vi "ModeMgr.Init.vi"(6 "Default Config File":path=path "C:/MTE/Facility/Modes.json", 8 "error in (no error)":errorcluster, 9 "ControlRef":refnum<vi>, 10 "Config File":path=path "C:/MTE/Facility/Modes.json", 11 "ModeMgr In":refnum<class "Mode Manager.lvclass">) -> (0 "error out":errorcluster, 1 "Mode Settings":T1[](array[typedef]), 2 "Mode":string, 3 "ModeMgr Out":refnum<class "Mode Manager.lvclass">)   [LabVIEW 2018, in "Mode Manager.lvclass"]
uses:
  Mode Manager.lvclass
  ModeMgr.Mode Settings.ctl
  Mode Manager.lvclass/Mode Manager.ctl
  <vilib>/KATE/Files/File Utils.lvlib
panel:
  out "Used Default":bool
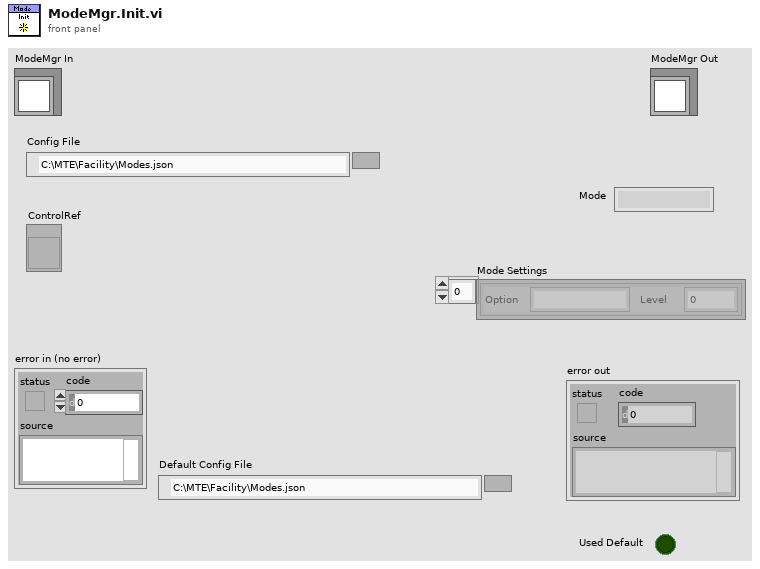
[diagram p1: front panel]
types:
  T1 = typedef "ModeMgr.Mode Settings.ctl" = cluster{"Option":string, "Level":i32}
  T2 = enum16{"open", "replace", "create", "open or create", "replace or create", "replace or create with confirmation"}
  T3 = typedef "ModeMgr.ModeConfig.ctl" = cluster{"Name":string, "Color":string, "Settings":T1[], "Password":string}
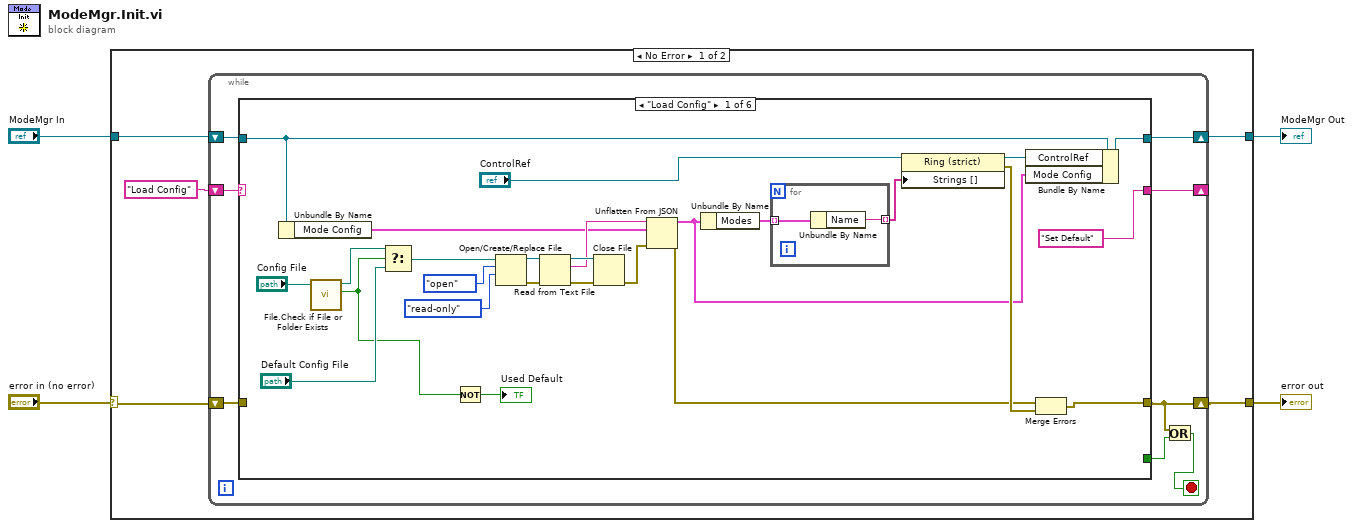
[diagram p0: block diagram]
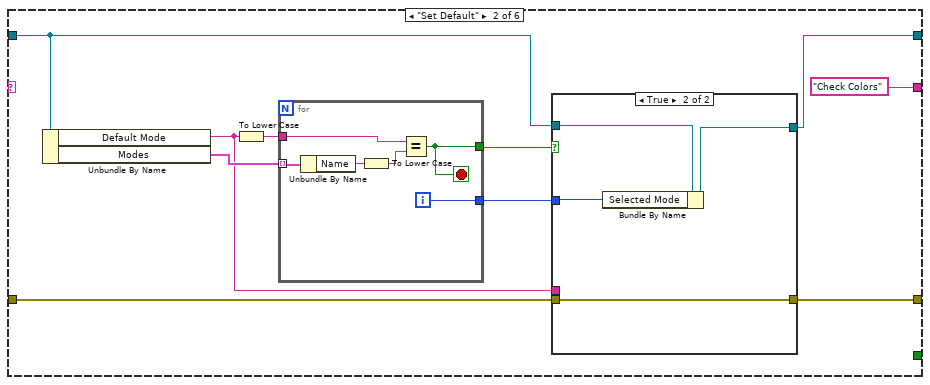
[diagram p2: hidden frame]
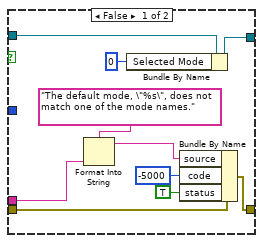
[diagram p3: hidden frame]
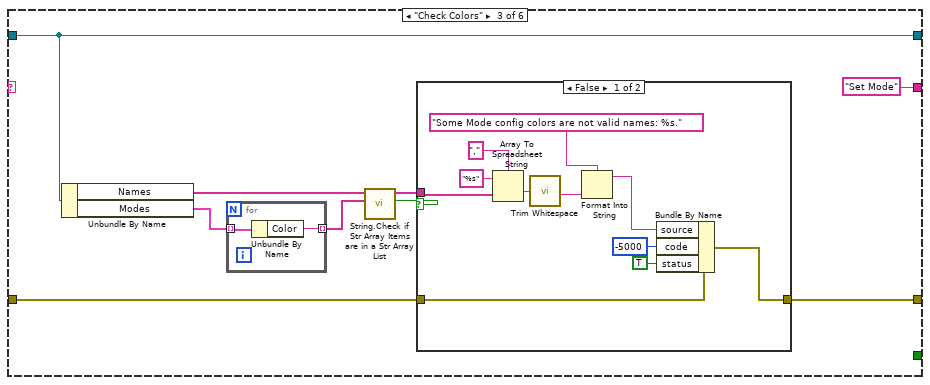
[diagram p4: hidden frame]
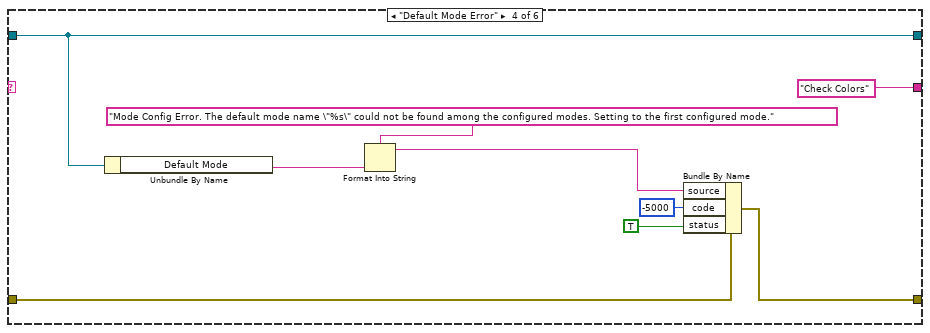
[diagram p6: hidden frame]
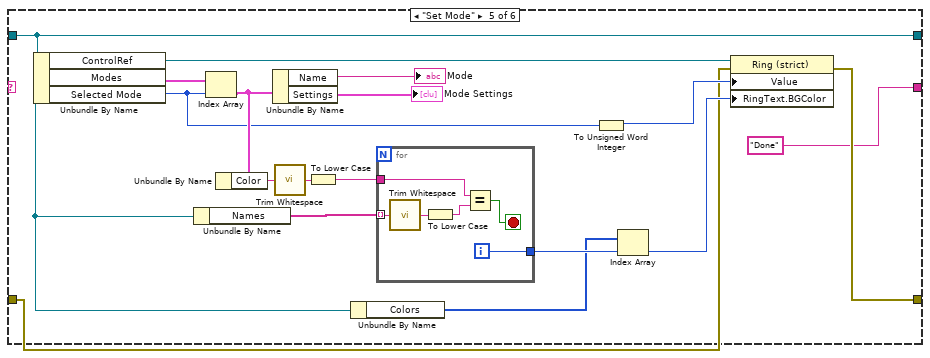
[diagram p7: hidden frame]
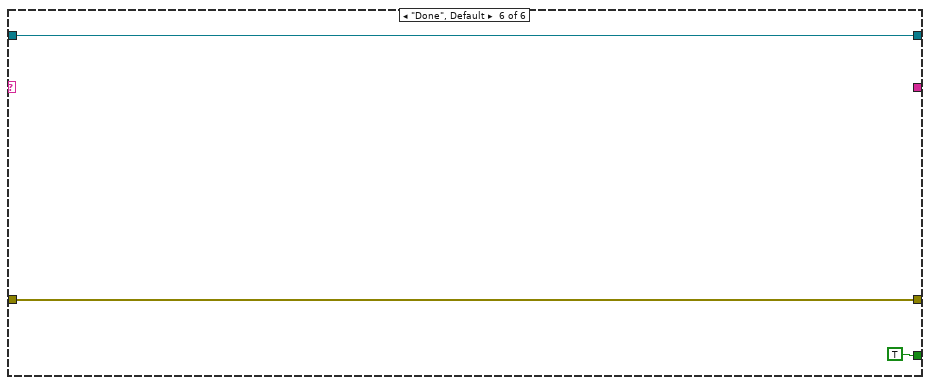
[diagram p8: hidden frame]
diagram:
  n1 = case shown="No Error" "error in (no error)" {
    selector: "error in (no error)" -> [w7 w136]
    tunnel: [w5 w136] -> w3
    tunnel: [w8 w135] -> w1
    tunnel: "ModeMgr In" -> [w9 w135]
    frame No Error {
      n2 = while {
        shift-right: [w16] -> w8
        shift-left: w9 -> [w17]
        shift-right: [w12] -> w5
        shift-left: w7 -> [w13]
        shift-right: [w14] -> _
        shift-left: "Load Config" -> [w15]
        stop <- w11 stop-if-true
        n3 = case shown="\"Load Config\"" w15 {
          tunnel: w17 -> [w36 w50 w78 w100 w115 w134]
          tunnel: [w35 w51 w78 w100 w115 w134] -> w16
          tunnel: [w29 w46 w76 w101 w113 w133] -> w12
          tunnel: ["Set Default" "Check Colors" "Set Mode" "Check Colors" "Done" _] -> w14
          tunnel: w13 -> [_ w48 w79 w102 w114 w133]
          tunnel: [_ _ _ _ _ TRUE] -> w10
          frame "Load Config" {
            n4 = Unbundle By Name(w36) -> ("Mode Config"=w27:cluster{"Default Mode":string, "Modes":T3[]})
            n5 = call <vilib>:"File.Check if File or Folder Exists.vi"("Path"="Config File") -> ("Exists"=w18:bool, "Dup Path"=w21:path)  [unwired: 6 in, 3 out]
            n6 = Select(t=w21, s=w18, f="Default Config File") -> (s? t:f=w22:path)
            n7 = Not(x=w18) -> (.not. x?=→"Used Default":bool)
            n8 = Open/Create/Replace File(file path (use dialog)=w22, operation (0:open)=T2."open", access (0:read/write)=enum16{"read/write", "read-only", "write-only"}."read-only") -> (refnum out=w42:refnum<file>, error out=w43:errorcluster)  [unwired: 3 in, 1 out]
            n9 = Read from Text File(file (use dialog)=w42, error in=w43) -> (refnum out=w41:refnum<file>, text=w37:string, error out=w40:errorcluster)  [unwired: 2 in, 1 out]
            n10 = Close File(refnum=w41, error in=w40) -> (error out=w34:errorcluster)  [unwired: 1 out]
            n11 = Unflatten From JSON(JSON string=w37, type and defaults=w27, error in (no error)=w34) -> (value=w24:cluster{"Default Mode":string, "Modes":T3[]}, error out=w28:errorcluster)  [unwired: 4 in]
            n12 = Unbundle By Name(w24) -> ("Modes"=w26:T3[])
            n13 = for {
              tunnel: w26 -> [w45] mode=indexing
              tunnel: [w44] -> w25 mode=indexing
              n14 = Unbundle By Name(w45) -> ("Name"=w44:string)
            }
            n15 = property class="Ring (strict)"(reference="ControlRef", "Strings []"=w25) -> (reference out=w32:refnum<vi>, error out=w30:errorcluster)  [unwired: 1 in]
            n16 = Bundle By Name(cluster=w36, "ControlRef"=w32, "Mode Config"=w24) -> (w35:refnum<class "Mode Manager.lvclass">)
            n17 = Merge Errors(w28, w30) -> (w29:errorcluster)
          }
          frame "Set Default" {
            n18 = Unbundle By Name(w50) -> ("Default Mode"=w47:string, "Modes"=w55:T3[])
            n19 = To Lower Case(string=w47) -> (all lower case string=w54:string)
            n20 = for {
              tunnel: w55 -> [w72] mode=indexing
              tunnel: w54 -> [w73]
              tunnel: [w71] -> w53
              tunnel: [w70] -> w52
              i -> [w70]
              stop <- w71 stop-if-true
              n21 = Unbundle By Name(w72) -> ("Name"=w74:string)
              n22 = To Lower Case(string=w74) -> (all lower case string=w75:string)
              n23 = Equal?(x=w73, y=w75) -> (x = y?=w71:bool)
            }
            n24 = case shown="True" w53 {
              tunnel: w52 -> [_ w67]
              tunnel: w50 -> [w65 w69]
              tunnel: [w64 w68] -> w51
              tunnel: w48 -> [w60 w66]
              tunnel: w47 -> [w61 _]
              tunnel: [w56 w66] -> w46
              frame False {
                n25 = Format Into String(format string="The default mode, \"%s\", does not match one of the mode names.", w61) -> (resulting string=w58:string)  [unwired: 2 in, 1 out]
                n26 = Bundle By Name(cluster=w65, "Selected Mode"=0) -> (w64:refnum<class "Mode Manager.lvclass">)
                n27 = Bundle By Name(cluster=w60, "source"=w58, "code"=-5000, "status"=TRUE) -> (w56:errorcluster)
              }
              frame True {
                n28 = Bundle By Name(cluster=w69, "Selected Mode"=w67) -> (w68:refnum<class "Mode Manager.lvclass">)
              }
            }
          }
          frame "Check Colors" {
            n29 = Unbundle By Name(w78) -> ("Names"=w84:string[], "Modes"=w83:T3[])
            n30 = for {
              tunnel: w83 -> [w98] mode=indexing
              tunnel: [w97] -> w82 mode=indexing
              n31 = Unbundle By Name(w98) -> ("Color"=w97:string)
            }
            n32 = call "String.Check if Str Array Items are in a Str Array List.vi"("Items to Check"=w82, "List"=w84) -> ("All Items in list"=w81:bool, "Items Not in List"=w80:string[])  [unwired: 7 in, 1 out]
            n33 = case shown="False" w81 {
              tunnel: w80 -> [w95 _]
              tunnel: w79 -> [w91 w96]
              tunnel: [w89 w96] -> w76
              frame False {
                n34 = Array To Spreadsheet String(delimiter (Tab)=",", array=w95, 3:"%s" ("format string")) -> (spreadsheet string=w85:string)
                n35 = call <vilib>:"Trim Whitespace.vi"("string"=w85) -> ("trimmed string"=w86:string)  [unwired: 1 in]
                n36 = Format Into String(format string="Some Mode config colors are not valid names: %s." ("delimiter (Tab)"), w86) -> (resulting string=w90:string)  [unwired: 2 in, 1 out]
                n37 = Bundle By Name(cluster=w91, "source"=w90, "code"=-5000, "status"=TRUE) -> (w89:errorcluster)
              }
              frame True {
                # "OK"
              }
            }
          }
          frame "Default Mode Error" {
            n38 = Unbundle By Name(w100) -> ("Default Mode"=w104:string)
            n39 = Format Into String(format string="Mode Config Error. The default mode name \"%s\" could not be found among the configured modes. Setting to the first configured mode.", w104) -> (resulting string=w103:string)  [unwired: 2 in, 1 out]
            n40 = Bundle By Name(cluster=w102, "source"=w103, "code"=-5000, "status"=TRUE) -> (w101:errorcluster)
          }
          frame "Set Mode" {
            n41 = Unbundle By Name(w115) -> ("ControlRef"=w120:refnum<vi>, "Modes"=w125:T3[], "Selected Mode"=w109:i32)
            n42 = Unbundle By Name(w115) -> ("Names"=w124:string[])
            n43 = Index Array(array=w125, index=w109) -> (element=w111:T3)
            n44 = Unbundle By Name(w111) -> ("Color"=w123:string)
            n45 = Unbundle By Name(w111) -> ("Name"=→"Mode":string, "Settings"=→"Mode Settings":T1[])
            n46 = call <vilib>:"Trim Whitespace.vi"("string"=w123) -> ("trimmed string"=w122:string)  [unwired: 1 in]
            n47 = To Lower Case(string=w122) -> (all lower case string=w121:string)
            n48 = Unbundle By Name(w115) -> ("Colors"=w118:u32[])
            n49 = for {
              tunnel: w124 -> [w130] mode=indexing
              tunnel: w121 -> [w128]
              tunnel: [w126] -> w119
              i -> [w126]
              stop <- w127 stop-if-true
              n50 = call <vilib>:"Trim Whitespace.vi"("string"=w130) -> ("trimmed string"=w131:string)  [unwired: 1 in]
              n51 = To Lower Case(string=w131) -> (all lower case string=w129:string)
              n52 = Equal?(x=w128, y=w129) -> (x = y?=w127:bool)
            }
            n53 = To Unsigned Word Integer(number=w109) -> (unsigned 16bit integer=w117:u16)
            n54 = Index Array(array=w118, index=w119) -> (element=w116:u32)
            n55 = property class="Ring (strict)"(reference=w120, error in=w114, "Value"=w117, "RingText.BGColor"=w116) -> (error out=w113:errorcluster)  [unwired: 1 out]
          }
          frame "Done", Default {
          }
        }
        n56 = Or(x=w12, y=w10) -> (x .or. y?=w11:bool)
      }
    }
    frame Error {
    }
  }
  "error out" <- w3
  "ModeMgr Out" <- w1
